vi "Write Pulse Enable.vi"(8 "error in":errorcluster, 10 "Chan_Trig_En":bool[](array[boolean]), 11 "Electronic Load in":refnum<class "Electronic Load.lvclass">) -> (0 "error out":errorcluster, 3 "Electronic Load out":refnum<class "Electronic Load.lvclass">)   [LabVIEW 2019, in "Electronic Load.lvlib" / "Electronic Load.lvclass"]
uses:
  Library/Electronic Load.lvclass
  C:/Users/Public/Documents/Development/builds/Instruments/Instruments.lvlibp/Library/Instruments.lvclass
  Library/Electronic Load.lvclass/Electronic Load.ctl
  builds/Instruments/Instruments.lvlibp/Private/Polymorphic/Special/Event from String.vi
  builds/Instruments/Instruments.lvlibp/Accessors/Command with Logging.vi
  builds/Instruments/Instruments.lvlibp/Library/Instruments.lvclass
  builds/Instruments/Instruments.lvlibp
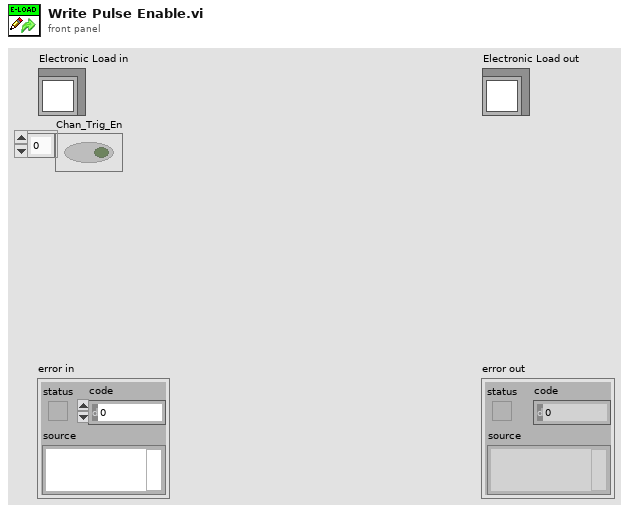
[diagram p1: front panel]
types:
  T1 = cluster{"Timestamp":timestamp, "Description":string, "Data":string}
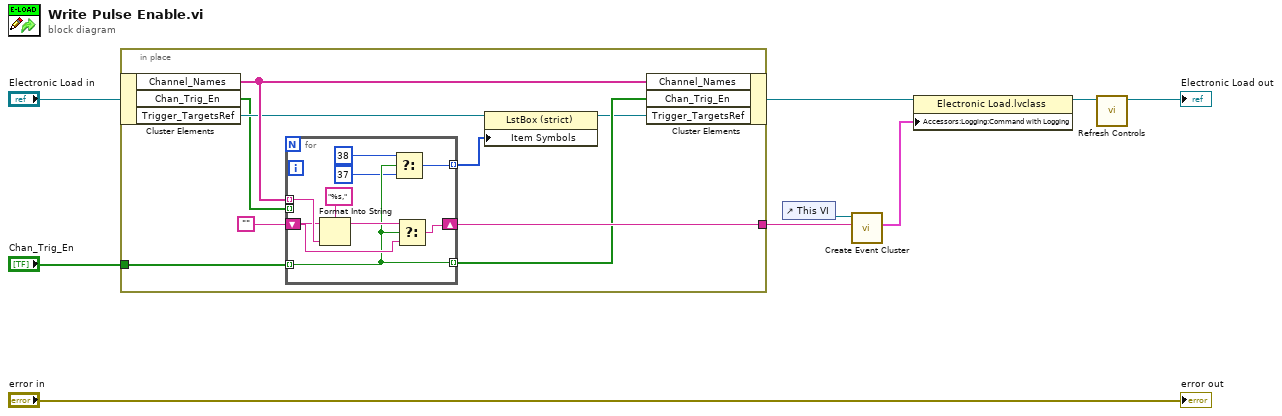
[diagram p0: block diagram]
diagram:
  n1 = in-place {
    in-place-border: "Chan_Trig_En" -> [w18]
    in-place-border: [w16] -> w5
    n2 = in-place-cluster #1("Electronic Load in") -> ("Channel_Names"=w15:string[], "Chan_Trig_En"=w10:bool[], "Trigger_TargetsRef"=w12:refnum<vi>)
    n3 = for {
      tunnel: w15 -> [w26] mode=indexing
      tunnel: w18 -> [w21] mode=indexing
      tunnel: [w21] -> w14 mode=indexing
      shift-right: [w27] -> w16
      shift-left: "" -> [w23]
      tunnel: [w19] -> w11 mode=indexing
      tunnel: w10 -> [_] mode=indexing
      n4 = Format Into String(format string="%s,", initial string=w23, w26) -> (resulting string=w24:string)  [unwired: 1 in, 1 out]
      n5 = Select(t=38, s=w21, f=37) -> (s? t:f=w19:i32)
      n6 = Select(t=w24, s=w21, f=w23) -> (s? t:f=w27:string)
    }
    n7 = property class="LstBox (strict)"(reference=w12, "Item Symbols"=w11) -> (reference out=w13:refnum<vi>)  [unwired: 1 in, 1 out]
    n8 = in-place-cluster #1("Channel_Names"=w15, "Chan_Trig_En"=w14, "Trigger_TargetsRef"=w13) -> (w3:refnum<class "Electronic Load.lvclass">)
  }
  n9 = control-ref of="This VI"() -> (w8:refnum<vi>)
  n10 = call-poly "Create Event Cluster.vi"("Value"=w5, "VI Refnum"=w8) -> ("Event Data"=w7:T1)  [unwired: 9 in]
  n11 = property class="Electronic Load.lvclass"(reference=w3, "Accessors:Logging:Command with Logging"=w7) -> (reference out=w2:refnum<class "Electronic Load.lvclass">)  [unwired: 1 in, 1 out]
  n12 = call "Refresh Controls.vi"("Electronic Load in"=w2) -> ("Electronic Load out"=→"Electronic Load out":refnum<class "Electronic Load.lvclass">)  [unwired: 9 in, 1 out]
  "error out" <- "error in"
